vi "Configure Temperature RTD.vi"(0 "VISA resource name":refnum<visa-resource-name>, 5 "Wire Mode (1: 4-Wire)":i16(ring)=1 items=["2-Wire", "4-Wire"], 7 "Unit (0: Celsius)":u16(ring) items=["C", "F", "K"], 9 "RTD Type (0: PT100_385)":u16(ring) items=["PT100_385", "PT100_392", "Custom"], 11 "error in (no error)":errorcluster, 12 "R0 (100 ohms)":i32=100, 13 "Alpha (385)":dbl=385.0 min=374.0 max=393.0 format="%#.6p") -> (4 "VISA resource name out":refnum<visa-resource-name>, 15 "error out":errorcluster)   [LabVIEW 2010, in "Fluke 884X Series.lvlib"]
doc: "Configures the settings for a 2-wire or 4-wire RTD probe.\n\n<B>Note:</B>\n\nThis VI only applies to the Fluke 8846A"
uses:
  <instrlib>/Fluke 884X Series/Fluke 884X Series.lvlib
panel:
  # "Custom RTD Type"
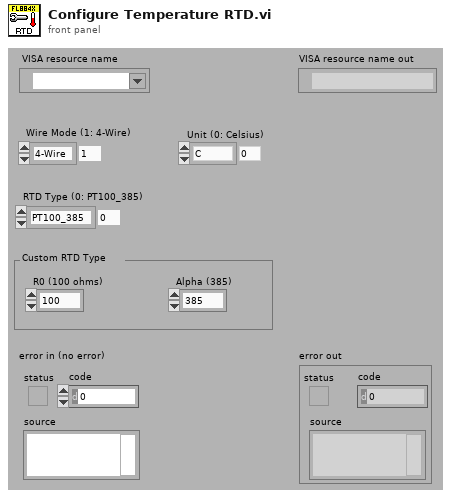
[diagram p1: front panel]
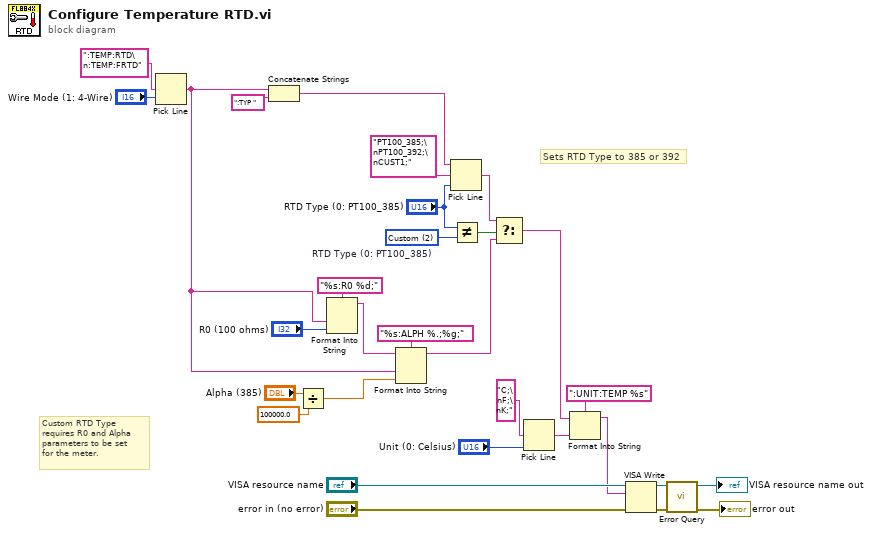
[diagram p0: block diagram]
diagram:
  w18 = u16 2 items=["PT100_385", "PT100_392", "Custom"]  # RTD Type (0: PT100_385)
  # "Custom RTD Type\nrequires R0 and Alpha\nparameters to be set \nfor the meter."
  # "Sets RTD Type to 385 or 392"
  n1 = Pick Line(multi-line string=":TEMP:RTD\n:TEMP:FRTD", line index="Wire Mode (1: 4-Wire)") -> (output string=w5:string)  [unwired: 1 in]
  n2 = Concatenate Strings(w5, ":TYP " ("string")) -> (w15:string)
  n3 = Divide(x="Alpha (385)", y=100000.0) -> (x/y=w9:dbl)
  n4 = Format Into String(format string="%s:R0 %d;", w5, "R0 (100 ohms)") -> (resulting string=w14:string)  [unwired: 2 in, 1 out]
  n5 = Format Into String(format string="%s:ALPH %.;%g;", initial string=w14, w5, w9) -> (resulting string=w7:string)  [unwired: 1 in, 1 out]
  n6 = Pick Line(string ("")=w15, multi-line string="PT100_385;\nPT100_392;\nCUST1;", line index="RTD Type (0: PT100_385)") -> (output string=w8:string)
  n7 = Not Equal?(x="RTD Type (0: PT100_385)", y=w18) -> (x != y?=w17:bool)
  n8 = Select(t=w8, s=w17, f=w7) -> (s? t:f=w2:string)
  n9 = Pick Line(multi-line string="C;\nF;\nK;", line index="Unit (0: Celsius)") -> (output string=w1:string)  [unwired: 1 in]
  n10 = Format Into String(format string=":UNIT:TEMP %s", initial string=w2, w1) -> (resulting string=w3:string)  [unwired: 1 in, 1 out]
  n11 = VISA Write(VISA resource name="VISA resource name", write buffer=w3, error in (no error)="error in (no error)") -> (VISA resource name out=w28:refnum<visa-resource-name>, error out=w27:errorcluster)  [unwired: 1 out]
  n12 = call <instrlib>:"Error Query.vi"("error in (no error)"=w27, "VISA resource name"=w28) -> ("error out"=→"error out":errorcluster, "VISA resource name out"=→"VISA resource name out":refnum<visa-resource-name>)  [unwired: 6 in, 2 out]
